vi "to Line Protocol.vi"(8 "error in":errorcluster, 10 "Use Timestamp?":bool, 11 "Data Point":T1 {"Time Stamp" format="%<%x %.3X>T"}) -> (0 "error out":errorcluster, 3 "Line Protocol":string)   [LabVIEW 2020, in "InfluxDB v2 Client.lvlib"]
doc: "Converts a data point into line protocol"
uses:
  InfluxDB v2 Client.lvlib
  Data Point.ctl
  Tag.ctl
  Field.ctl
  Timestamp precision.ctl
panel:
  # "to Line Protocol.vi"
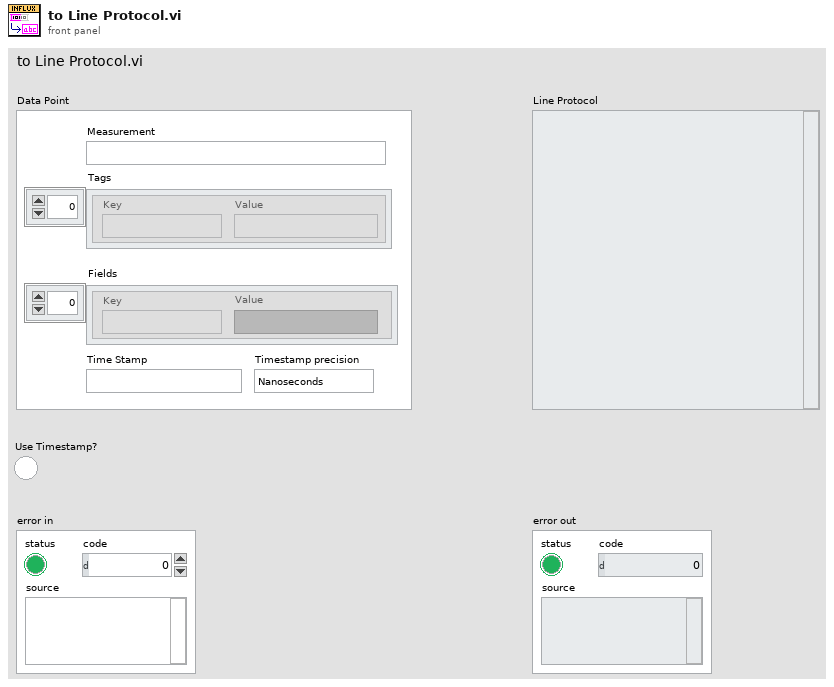
[diagram p1: front panel]
types:
  T1 = typedef "InfluxDB v2 Client.lvlib/Data Point.ctl" = cluster{"Measurement":string, "Tags":T2[], "Fields":T3[], "Timestamp precision":T4, "Time Stamp":timestamp}
  T2 = typedef "InfluxDB v2 Client.lvlib/Tag.ctl" = cluster{"Key":string, "Value":string}
  T3 = typedef "InfluxDB v2 Client.lvlib/Field.ctl" = cluster{"Key":string, "Value":variant}
  T4 = typedef "InfluxDB v2 Client.lvlib/Timestamp precision.ctl" = enum16{"Nanoseconds", "Microseconds", "Milliseconds", "Seconds"}
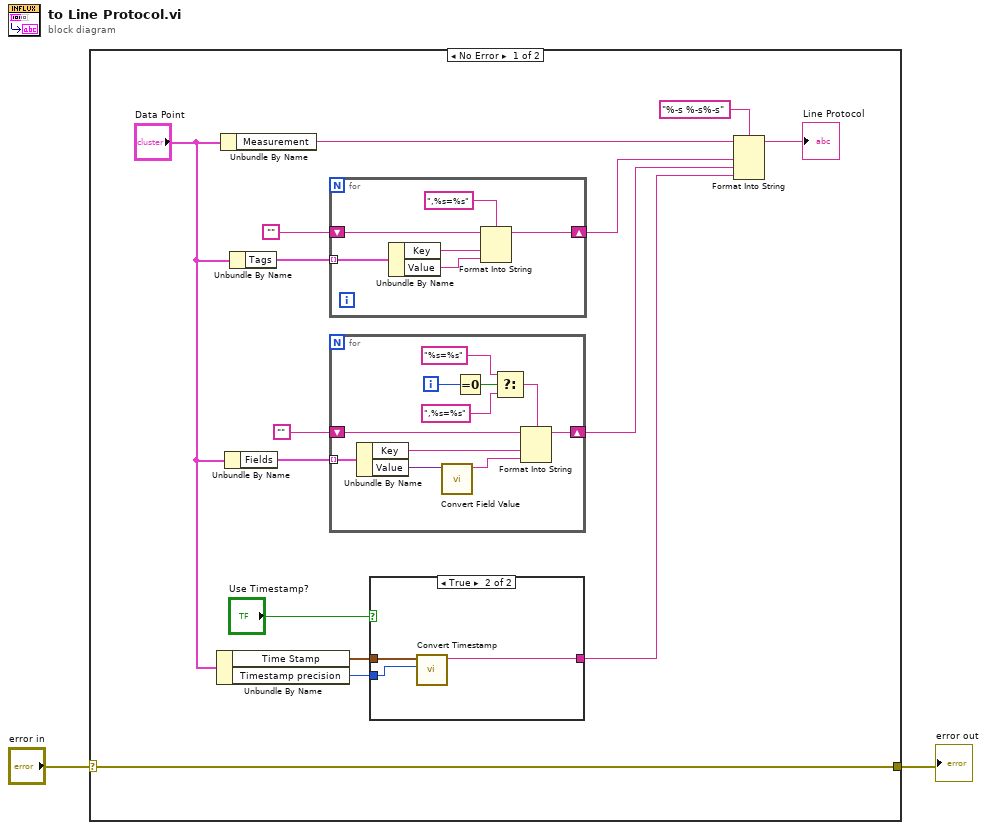
[diagram p0: block diagram]
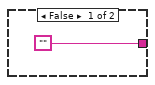
[diagram p2: hidden frame]
diagram:
  n1 = case shown="No Error" "error in" {
    selector: "error in" -> [w17 w39]
    tunnel: [w17 w39] -> w1
    frame No Error {
      n2 = Unbundle By Name("Data Point") -> ("Time Stamp"=w5:timestamp, "Timestamp precision"=w4:T4)
      n3 = Unbundle By Name("Data Point") -> ("Measurement"=w16:string)
      n4 = Unbundle By Name("Data Point") -> ("Fields"=w10:T3[])
      n5 = Unbundle By Name("Data Point") -> ("Tags"=w13:T2[])
      n6 = for {
        tunnel: w13 -> [w38] mode=indexing
        shift-right: [w35] -> w11
        shift-left: "" -> [w36]
        n7 = Unbundle By Name(w38) -> ("Key"=w34:string, "Value"=w33:string)
        n8 = Format Into String(format string=",%s=%s", initial string=w36, w34, w33) -> (resulting string=w35:string)  [unwired: 1 in, 1 out]
      }
      n9 = for {
        tunnel: w10 -> [w32] mode=indexing
        shift-right: [w30] -> w9
        shift-left: "" -> [w31]
        i -> [w26]
        n10 = Unbundle By Name(w32) -> ("Key"=w29:string, "Value"=w28:variant)
        n11 = call "Convert Field Value.vi"("Field Value"=w28) -> ("Field String"=w27:string)  [unwired: 9 in, 1 out]
        n12 = Equal To 0?(x=w26) -> (x = 0?=w25:bool)
        n13 = Select(t="%s=%s" ("format string"), s=w25, f=",%s=%s" ("format string")) -> (s? t:f=w22:string)
        n14 = Format Into String(format string=w22, initial string=w31, w29, w27) -> (resulting string=w30:string)  [unwired: 1 in, 1 out]
      }
      n15 = case shown="True" "Use Timestamp?" {
        tunnel: w5 -> [_ w21]
        tunnel: w4 -> [_ w20]
        tunnel: ["" w19] -> w3
        frame False {
        }
        frame True {
          n16 = call "Convert Timestamp.vi"("Timestamp precision"=w20, "Time Stamp"=w21) -> ("Timestamp String"=w19:string)  [unwired: 9 in]
        }
      }
      n17 = Format Into String(format string="%-s %-s%-s", initial string=w16, w11, w9, w3) -> (resulting string=→"Line Protocol":string)  [unwired: 1 in, 1 out]
    }
    frame Error {
    }
  }
  "error out" <- w1
